vi "Stack PID Fan.vi"(6 "Reinitialize":bool, 10 "Temperature":dbl) -> (3 "Output":dbl)   [LabVIEW 2024]
uses:
  <vilib>/addons/control/pid/NI_PID_pid.lvlib
  <vilib>/addons/control/pid/pid.llb/PID (DBL).vi
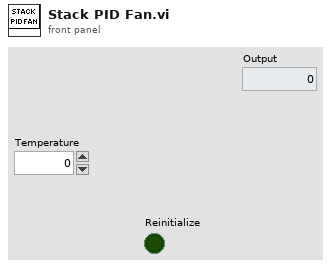
[diagram p1: front panel]
types:
  T1 = cluster{"proportional gain (Kc)":dbl, "integral time (Ti, min)":dbl, "derivative time (Td, min)":dbl}
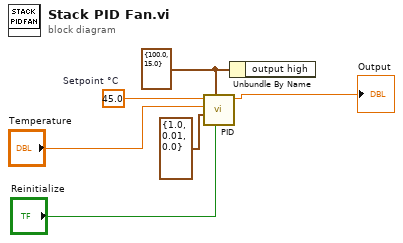
[diagram p0: block diagram]
diagram:
  w5 = 45.0  # Setpoint °C
  w4 = cluster{"output high":dbl, "output low":dbl} {"output high"=100.0, "output low"=15.0} ("output range")
  n1 = call-poly <vilib>:"PID.vi"("reinitialize? (F)"="Reinitialize", "output range"=w4, "PID gains"=T1 {"proportional gain (Kc)"=1.0, "integral time (Ti, min)"=0.01, "derivative time (Td, min)"=0.0}, "process variable"="Temperature", "setpoint"=w5) -> ("output"=→"Output":dbl)  [unwired: 5 in, 1 out]
  n2 = Unbundle By Name(w4) -> ()  [unwired: 1 out]
